vi "Auto 3.vi"(8 "Error In":errorcluster) -> ()   [LabVIEW 2014]
uses:
  Robot Global Data.vi
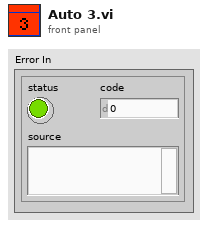
[diagram p1: front panel]
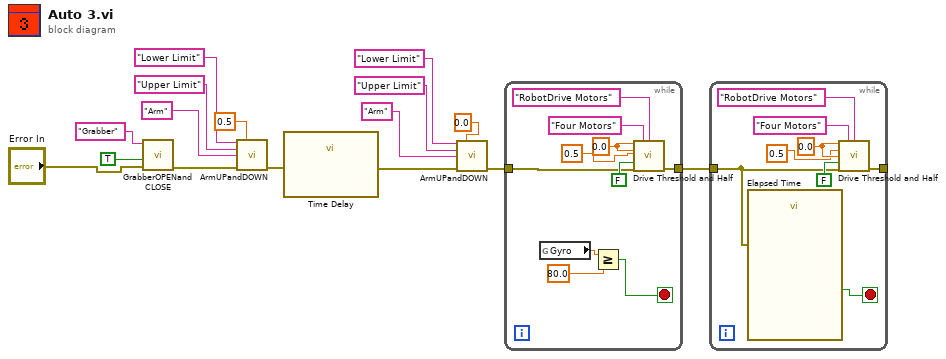
[diagram p0: block diagram]
diagram:
  n1 = call "GrabberOPENandCLOSE.vi"("Error In"="Error In", "Grabber Open/Close"=TRUE, "refnum name"="Grabber") -> ("Error Out"=w8:errorcluster)  [unwired: 8 in]
  n2 = call "ArmUPandDOWN.vi"("Lower Limit"="Lower Limit" ("refnum name"), "Arm Value"=0.5, "Upper Limit"="Upper Limit" ("refnum name"), "Arm"="Arm" ("refnum name"), "Error In"=w8) -> ("Error Out"=w10:errorcluster)  [unwired: 8 in, 2 out]
  n3 = call "Time Delay"("error in (no error)"=w10) -> ("error out"=w15:errorcluster)  [unwired: 10 in]
  n4 = call "ArmUPandDOWN.vi"("Lower Limit"="Lower Limit" ("refnum name"), "Arm Value"=0.0, "Upper Limit"="Upper Limit" ("refnum name"), "Arm"="Arm" ("refnum name"), "Error In"=w15) -> ("Error Out"=w16:errorcluster)  [unwired: 8 in, 2 out]
  n5 = while {
    tunnel: w16 -> [w23]
    tunnel: [w22] -> w1
    stop <- w17 stop-if-true
    w21 = 0.0 ("Arm Value")
    n6 = global read "Robot Global Data.vi" "Gyro"() -> (w19:dbl)
    n7 = Greater Or Equal?(x=w19, y=80.0) -> (x >= y?=w17:bool)
    n8 = call "Drive Threshold and Half.vi"("X In"=w21, "Drive refnum name"="Four Motors" ("refnum name"), "Send to DB Name"="RobotDrive Motors" ("Name"), "Y In"=w21, "R In"=0.5 ("X In"), "Speed Toggle"=FALSE ("Grabber Open/Close"), "Error In"=w23) -> ("Error Out"=w22:errorcluster)  [unwired: 8 in]
  }
  n9 = while {
    tunnel: w1 -> [w27]
    tunnel: [w31] -> _
    stop <- w28 stop-if-true
    w30 = 0.0 ("Arm Value")
    n10 = call "Elapsed Time"("error in (no error)"=w27) -> ("Time has Elapsed"=w28:bool)  [unwired: 11 in, 7 out]
    n11 = call "Drive Threshold and Half.vi"("X In"=w30, "Drive refnum name"="Four Motors" ("refnum name"), "Send to DB Name"="RobotDrive Motors" ("Name"), "Y In"=0.5 ("X In"), "R In"=w30, "Speed Toggle"=FALSE ("Grabber Open/Close"), "Error In"=w27) -> ("Error Out"=w31:errorcluster)  [unwired: 8 in]
  }
